vi "Manage DataPlugins.vi"() -> ()   [LabVIEW 2023]
doc: "This example demonstrates how to use the Manage DataPlugins VIs to create a DataPlugin Manager application. The DataPlugin Manager application lists all DataPlugins, including the name, type, file extensions, and version information, installed on the local computer when you first open this application. You can use this application to import, export, encrypt, or remove DataPlugins. \n\nImporting a DataPlugin registers the DataPlugin to the local computer. After you download a DataPlugin .uri file from the National Instruments Web site at ni.com/dataplugins, click the <B>Import</B> button to import the DataPlugin to the DataPlugin Manager. You then can use the DataPlugin to access the corresponding file format.\n\nExporting a DataPlugin enables you to generate a DataPlugin .uri file from a DataPlugin that you created in NI DIAdem. After you create a DataPlugin, the name and related information appears in the DataPlugin Manager. Select the DataPlugin and click the <B>Export</B> button to export the DataPlugin to a .uri file. You then can distribute the .uri file to other users. To export an encrypted DataPlugin, click the <B>Encrypt</B> button. Refer to ni.com/diadem for more information about NI DIAdem.\n\n\nRemoving a DataPlugin unregisters the DataPlugin from the local computer. Select the DataPlugin you want to remove and click the <B>Remove</B> button. This button does not delete the corresponding DataPlugin .uri file or installer from the computer.\n\n<B>Note:</B> DataPlugins are shared between different National Instruments products and applications on the local computer. Registering or unregistering a DataPlugin might affect these products or applications."
uses:
  <vilib>/Platform/storage/utility/Register DataPlugin by URI.vi
panel:
  in  "export prompt":string="Export a DataPlugin"
  in  "import prompt":string="Import a DataPlugin"
  in  "pattern label":string="DataPlugin File"
  in  "Encrypt":bool
  in  "Remove":bool
  in  "Export":bool
  in  "Stop":bool
  in  "Import":bool
  in  "DataPlugin Settings":i32(listbox)
  # "Overview: Demonstrates the use of the Manage DataPlugins VIs to configure the DataPlugins currently installed on this computer.\nRequirements: Windows\nInstructions:\n1. Run the VI.\n2. View the configuration information for all the DataPlugins currently installed on this computer.\n3. Experiment with importing, exporting, encrypting, and removing DataPlugins.\n4. Click Stop to stop the VI."
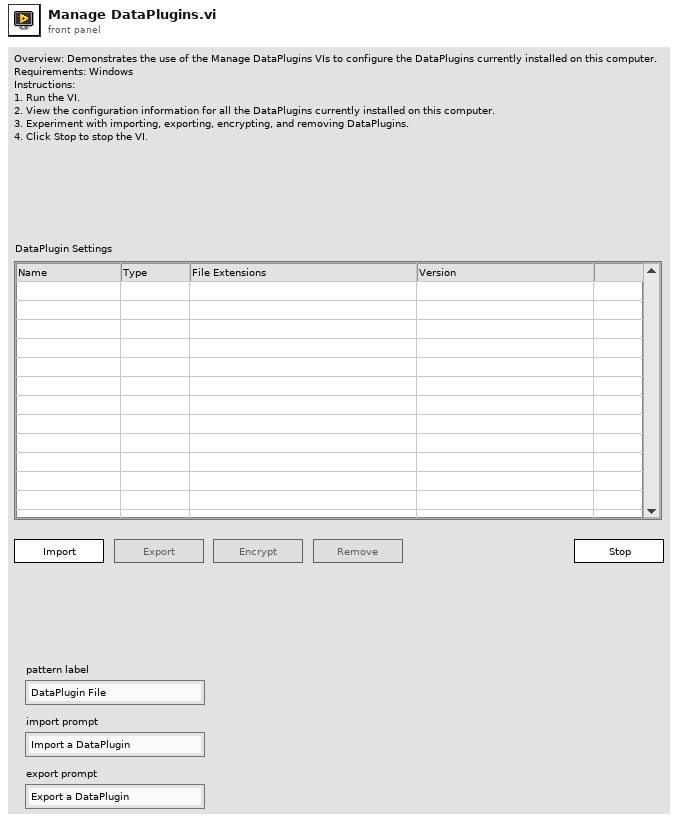
[diagram p1: front panel]
types:
  T1 = enum8{"Enabled", "Disabled", "Disabled and Grayed Out"}
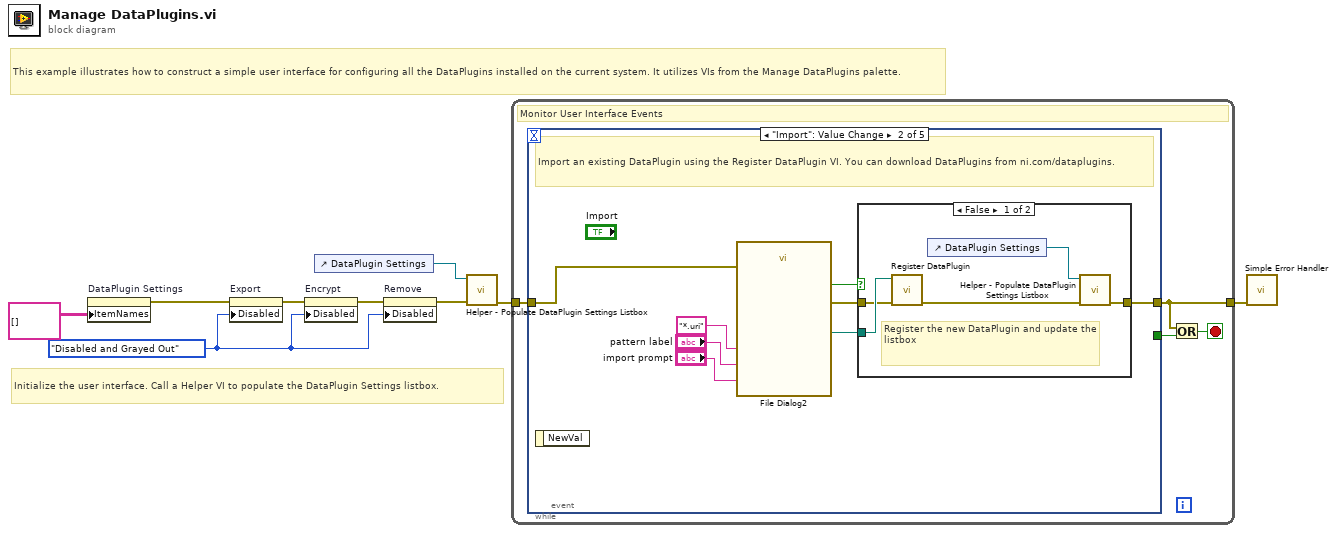
[diagram p0: block diagram]
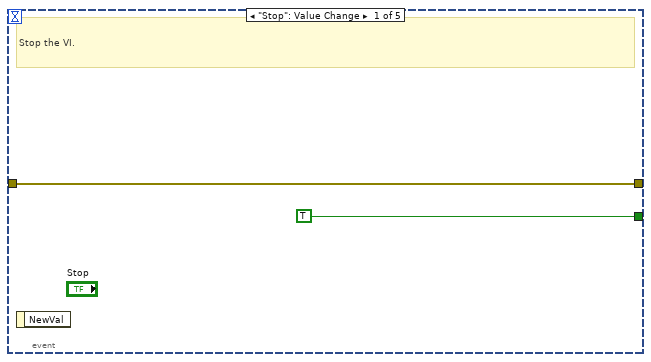
[diagram p2: hidden frame]
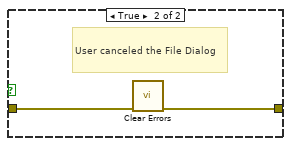
[diagram p3: hidden frame]
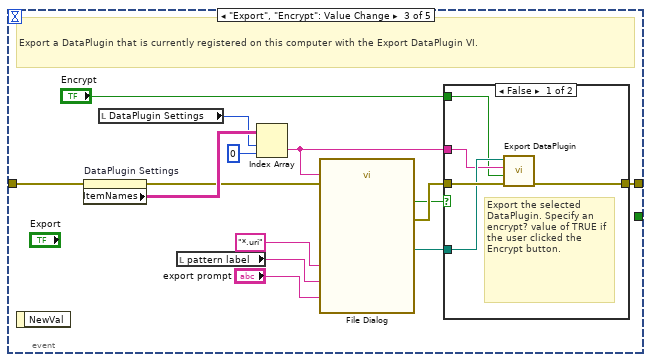
[diagram p4: hidden frame]
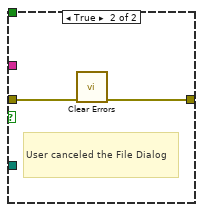
[diagram p5: hidden frame]
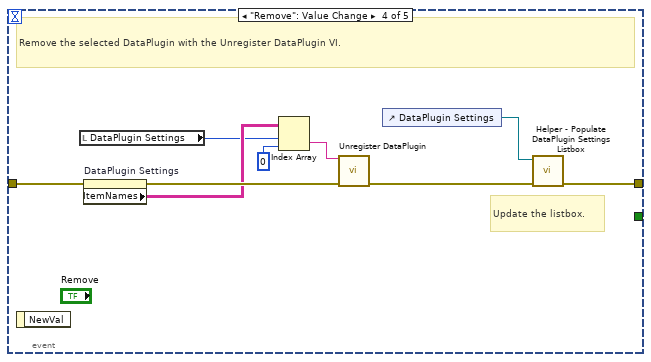
[diagram p6: hidden frame]
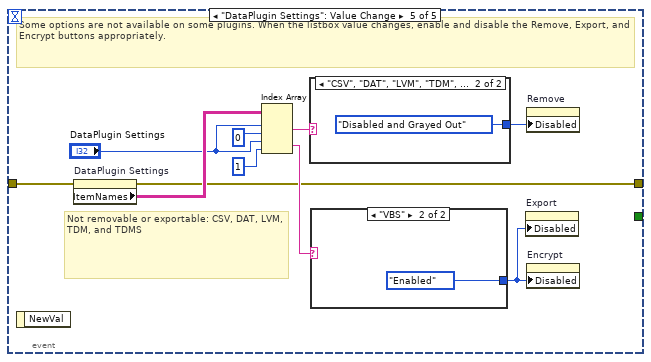
[diagram p7: hidden frame]
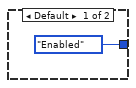
[diagram p8: hidden frame]
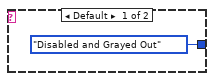
[diagram p9: hidden frame]
diagram:
  w6 = T1."Disabled and Grayed Out" ("Disabled")
  # "This example illustrates how to construct a simple user interface for configuring all the DataPlugins installed on the current system. It utilizes VIs from the Manage DataPlugins palette."
  # "Initialize the user interface. Call a Helper VI to populate the DataPlugin Settings listbox."
  n1 = property on="DataPlugin Settings" class="MCListbox (strict)"("ItemNames"=string[][] [] ("Item Names")) -> (error out=w3:errorcluster)  [unwired: 2 in, 1 out]
  n2 = property on="Export" class="Bool"(error in=w3, "Disabled"=w6) -> (error out=w7:errorcluster)  [unwired: 1 in, 1 out]
  n3 = property on="Encrypt" class="Bool"(error in=w7, "Disabled"=w6) -> (error out=w5:errorcluster)  [unwired: 1 in, 1 out]
  n4 = control-ref of="DataPlugin Settings"() -> (w1:refnum<vi>)
  n5 = property on="Remove" class="Bool"(error in=w5, "Disabled"=w6) -> (error out=w8:errorcluster)  [unwired: 1 in, 1 out]
  n6 = call "Helper - Populate DataPlugin Settings Listbox.vi"("error in (no error)"=w8, "DataPlugins Settings"=w1) -> ("error out"=w9:errorcluster)  [unwired: 9 in]
  n7 = while {
    tunnel: w9 -> [w13]
    tunnel: [w12] -> w4
    stop <- w11 stop-if-true
    # "Monitor User Interface Events"
    n8 = event shown="[1] \"Import\": Value Change" {
      selector: _ -> [_ _ _ _ _]
      dyn-events: _ -> [_ _ _ _ _]
      timeout: _ -> [_ _ _ _ _]
      tunnel: [TRUE _ _ _ _] -> w10
      tunnel: w13 -> [w14 w19 w38 w59 w70]
      tunnel: [w14 w23 w42 w53 w61] -> w12
      event "Stop": Value Change {
        # "Stop the VI."
        n9 = event-data() -> ()  [unwired: 2 out]
      }
      event "Import": Value Change {
        # "Import an existing DataPlugin using the Register DataPlugin VI. You can download DataPlugins from ni.com/dataplugins."
        n10 = event-data() -> ()  [unwired: 2 out]
        n11 = call "File Dialog2"("prompt"="import prompt", "error in"=w19, "pattern (all files)"="*.uri", "pattern label"="pattern label") -> ("selected path"=w22:path, "cancelled"=w20:bool, "error out"=w21:errorcluster)  [unwired: 8 in, 1 out]
        n12 = case shown="False" w20 {
          tunnel: [w24 w29] -> w23
          tunnel: w22 -> [w28 _]
          tunnel: w21 -> [w27 w30]
          frame False {
            # "Register the new DataPlugin and update the listbox"
            n13 = call-poly <vilib>:"Register DataPlugin.vi"("error in (no error)"=w27, "DataPlugin URI path (*.uri)"=w28) -> ("error out"=w25:errorcluster)  [unwired: 7 in, 2 out]
            n14 = control-ref of="DataPlugin Settings"() -> (w26:refnum<vi>)
            n15 = call "Helper - Populate DataPlugin Settings Listbox.vi"("error in (no error)"=w25, "DataPlugins Settings"=w26) -> ("error out"=w24:errorcluster)  [unwired: 9 in]
          }
          frame True {
            # "User canceled the File Dialog"
            n16 = call <vilib>:"Clear Errors.vi"("error in (no error)"=w30) -> ("error out"=w29:errorcluster)  [unwired: 5 in, 1 out]
          }
        }
      }
      event "Export", "Encrypt": Value Change {
        # "Export a DataPlugin that is currently registered on this computer with the Export DataPlugin VI."
        n17 = event-data() -> ()  [unwired: 2 out]
        n18 = property on="DataPlugin Settings" class="MCListbox (strict)"(error in=w38) -> (error out=w37:errorcluster, "ItemNames"=w44:string[][])  [unwired: 1 in, 1 out]
        n19 = local read "DataPlugin Settings"() -> (w35:i32)
        n20 = local read "pattern label"() -> (w34:string)
        n21 = Index Array(array=w44, index (row)=w35, index (col)=0 ("disabled index (col)")) -> (element=w39:string)
        n22 = call "File Dialog"("prompt"="export prompt", "default name"=w39, "error in"=w37, "pattern (all files)"="*.uri", "pattern label"=w34) -> ("selected path"=w40:path, "cancelled"=w36:bool, "error out"=w41:errorcluster)  [unwired: 7 in, 1 out]
        n23 = case shown="False" w36 {
          tunnel: [w49 w50] -> w42
          tunnel: w41 -> [w48 w51]
          tunnel: w40 -> [w47 _]
          tunnel: w39 -> [w46 _]
          tunnel: "Encrypt" -> [w45 _]
          frame False {
            # "Export the selected DataPlugin. Specify an encrypt? value of TRUE if the user clicked the Encrypt button."
            n24 = call <vilib>:"Export DataPlugin.vi"("error in (no error)"=w48, "encrypt? (F)"=w45, "DataPlugin name"=w46, "DataPlugin URI path (*.uri)"=w47) -> ("error out"=w49:errorcluster)  [unwired: 6 in, 1 out]
          }
          frame True {
            # "User canceled the File Dialog"
            n25 = call <vilib>:"Clear Errors.vi"("error in (no error)"=w51) -> ("error out"=w50:errorcluster)  [unwired: 5 in, 1 out]
          }
        }
      }
      event "Remove": Value Change {
        # "Update the listbox."
        # "Remove the selected DataPlugin with the Unregister DataPlugin VI."
        n26 = event-data() -> ()  [unwired: 2 out]
        n27 = local read "DataPlugin Settings"() -> (w55:i32)
        n28 = property on="DataPlugin Settings" class="MCListbox (strict)"(error in=w59) -> (error out=w58:errorcluster, "ItemNames"=w56:string[][])  [unwired: 1 in, 1 out]
        n29 = Index Array(array=w56, index (row)=w55, index (col)=0 ("disabled index (col)")) -> (element=w57:string)
        n30 = call <vilib>:"Unregister DataPlugin.vi"("DataPlugin name"=w57, "error in (no error)"=w58) -> ("error out"=w54:errorcluster)  [unwired: 13 in]
        n31 = control-ref of="DataPlugin Settings"() -> (w52:refnum<vi>)
        n32 = call "Helper - Populate DataPlugin Settings Listbox.vi"("error in (no error)"=w54, "DataPlugins Settings"=w52) -> ("error out"=w53:errorcluster)  [unwired: 9 in]
      }
      event "DataPlugin Settings": Value Change {
        # "Not removable or exportable: CSV, DAT, LVM, TDM, and TDMS"
        # "Some options are not available on some plugins. When the listbox value changes, enable and disable the Remove, Export, and Encrypt buttons appropriately."
        n33 = event-data() -> ()  [unwired: 2 out]
        n34 = property on="DataPlugin Settings" class="MCListbox (strict)"(error in=w70) -> (error out=w61:errorcluster, "ItemNames"=w67:string[][])  [unwired: 1 in, 1 out]
        n35 = Index Array(array=w67, index (row) #1="DataPlugin Settings", index (col) #1=0 ("disabled index (col)"), index (row) #2="DataPlugin Settings", index (col) #2=1 ("disabled index (col)")) -> (element #1=w66:string, element #2=w62:string)
        n36 = case shown="\"CSV\", \"DAT\", \"LVM\", \"TDM\", \"TDMS\"" w66 {
          tunnel: [T1."Enabled" ("Disabled") T1."Disabled and Grayed Out" ("Disabled")] -> w65
          frame Default {
          }
          frame "CSV", "DAT", "LVM", "TDM", "TDMS" {
          }
        }
        n37 = case shown="\"VBS\"" w62 {
          tunnel: [T1."Disabled and Grayed Out" ("Disabled") T1."Enabled" ("Disabled")] -> w69
          frame Default {
          }
          frame "VBS" {
          }
        }
        n38 = property on="Export" class="Bool"("Disabled"=w69) -> ()  [unwired: 2 in, 2 out]
        n39 = property on="Remove" class="Bool"("Disabled"=w65) -> ()  [unwired: 2 in, 2 out]
        n40 = property on="Encrypt" class="Bool"("Disabled"=w69) -> ()  [unwired: 2 in, 2 out]
      }
    }
    n41 = Or(x=w12, y=w10) -> (x .or. y?=w11:bool)
  }
  n42 = call <vilib>:"Simple Error Handler.vi"("error in (no error)"=w4) -> ()  [unwired: 4 in, 5 out]
